vi "T7_I2CWrite_UINT16_Register1.vi"(0 "Remote IP Address":string="192.168.126.148", 1 "Remote Port":u16=502, 2 "Starting Address":u16, 3 "error in (no error)":errorcluster, 4 "UINT16 to Write":u16) -> (9 "WrittenAt":timestamp=timestamp(3514396125.332373 s since 1904-01-01), 10 "error out":errorcluster)   [LabVIEW 2014]
uses:
  Serial Link Layer/NI_Modbus_Cleaned/NI Modbus121Clean.llb/MB Ethernet Master Query Write Multiple Registers (poly).vi
panel:
  # "MB Ethernet Example Master.vi\n\nInstructions\n1.Use Kipling to find your devices IP address & modify the\n\"Remote IP Addres\"\n2. Run this VI\n3. Change value of \"UINT16 to Write\" & press \"Write Data\""
  # "TCP Parameters"
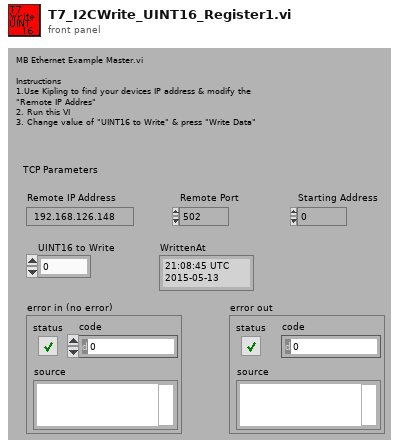
[diagram p1: front panel]
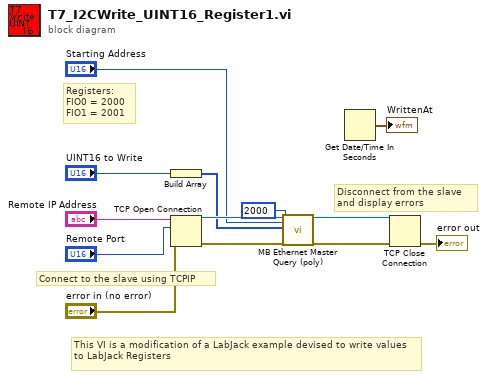
[diagram p0: block diagram]
diagram:
  # "This VI is a modification of a LabJack example devised to write values to LabJack Registers"
  # "Registers:\nFIO0 = 2000\nFIO1 = 2001"
  # "Disconnect from the slave\nand display errors"
  # "Connect to the slave using TCPIP"
  n1 = Build Array("UINT16 to Write") -> (w7:u16[])
  n2 = TCP Open Connection(address="Remote IP Address", remote port or service name="Remote Port", error in (no error)="error in (no error)") -> (connection ID=w11:refnum<k5>, error out=w10:errorcluster)  [unwired: 2 in]
  n3 = call-poly "MB Ethernet Master Query (poly).vi"("TCP Connection Refnum in"=w11, "Starting Address"="Starting Address", "Registers"=w7, "Timeout"=u32 2000, "error in"=w10) -> ("TCP Connection Refnum (dup)"=w9:refnum<k5>, "error out"=w8:errorcluster)  [unwired: 12 in, 1 out]
  n4 = Get Date/Time In Seconds() -> (seconds since 1Jan1904=→"WrittenAt":timestamp)
  n5 = TCP Close Connection(connection ID=w9, error in (no error)=w8) -> (error out=→"error out":errorcluster)  [unwired: 2 out]
